vi "validate inputs.vi"(9 "output in":T5, 10 "process in":T3, 11 "input in":T4) -> (3 "spec":T1[](array[typedef]))   [LabVIEW 2013, in "data interface script.lvlib"]
uses:
  data interface script.lvlib
  Controls/output script control.ctl
  Controls/input script control.ctl
  Controls/processing script control.ctl
  Controls/scripting spec.ctl
  <vilib>/NI/Tag Bus Module Framework/channel/channel classification.ctl
  <vilib>/NI/Tag Bus Module Framework/channel/TBM channel.lvclass
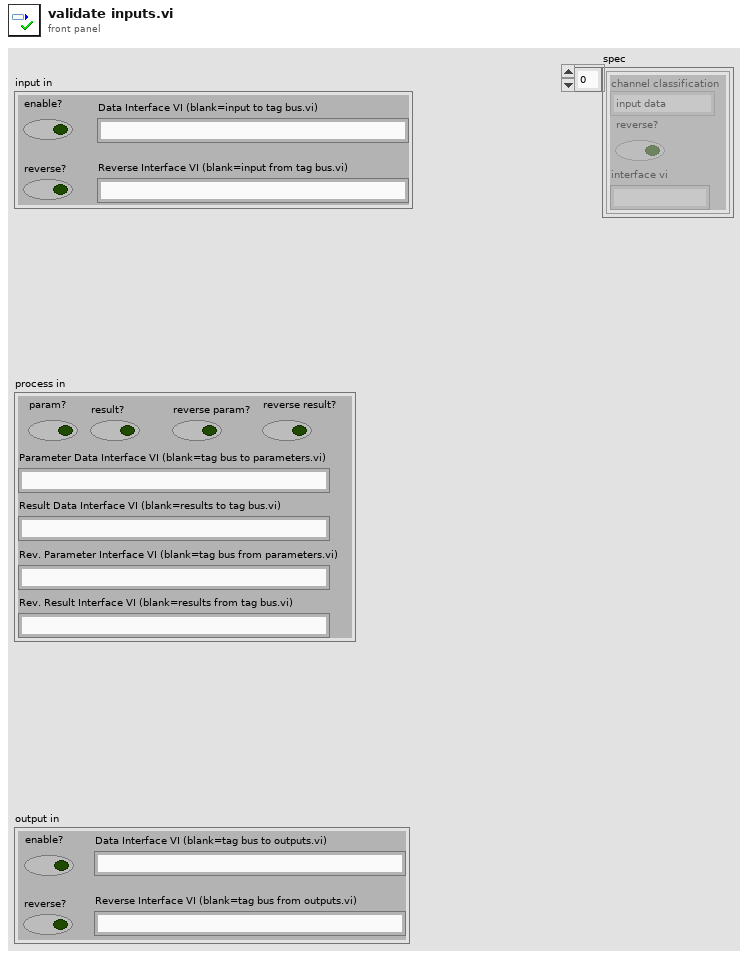
[diagram p1: front panel]
types:
  T1 = typedef "data interface script.lvlib/scripting spec.ctl" = cluster{"channel classification":T2, "reverse?":bool, "interface vi":string}
  T2 = typedef "TBM channel.lvclass/channel classification.ctl" = enum16{"input data", "output data", "processing parameter", "processing result"}
  T3 = typedef "data interface script.lvlib/processing script control.ctl" = cluster{"param?":bool, "Parameter Data Interface VI (blank=tag bus to parameters.vi)":string, "Result Data Interface VI (blank=results to tag bus.vi)":string, "reverse param?":bool, "Rev. Result Interface VI (blank=results from tag bus.vi)":string, "Rev. Parameter Interface VI (blank=tag bus from parameters.vi)":string, "result?":bool, "reverse result?":bool}
  T4 = typedef "data interface script.lvlib/input script control.ctl" = cluster{"enable?":bool, "Data Interface VI (blank=input to tag bus.vi)":string, "reverse?":bool, "Reverse Interface VI (blank=input from tag bus.vi)":string}
  T5 = typedef "data interface script.lvlib/output script control.ctl" = cluster{"enable?":bool, "Data Interface VI (blank=tag bus to outputs.vi)":string, "Reverse Interface VI (blank=tag bus from outputs.vi)":string, "reverse?":bool}
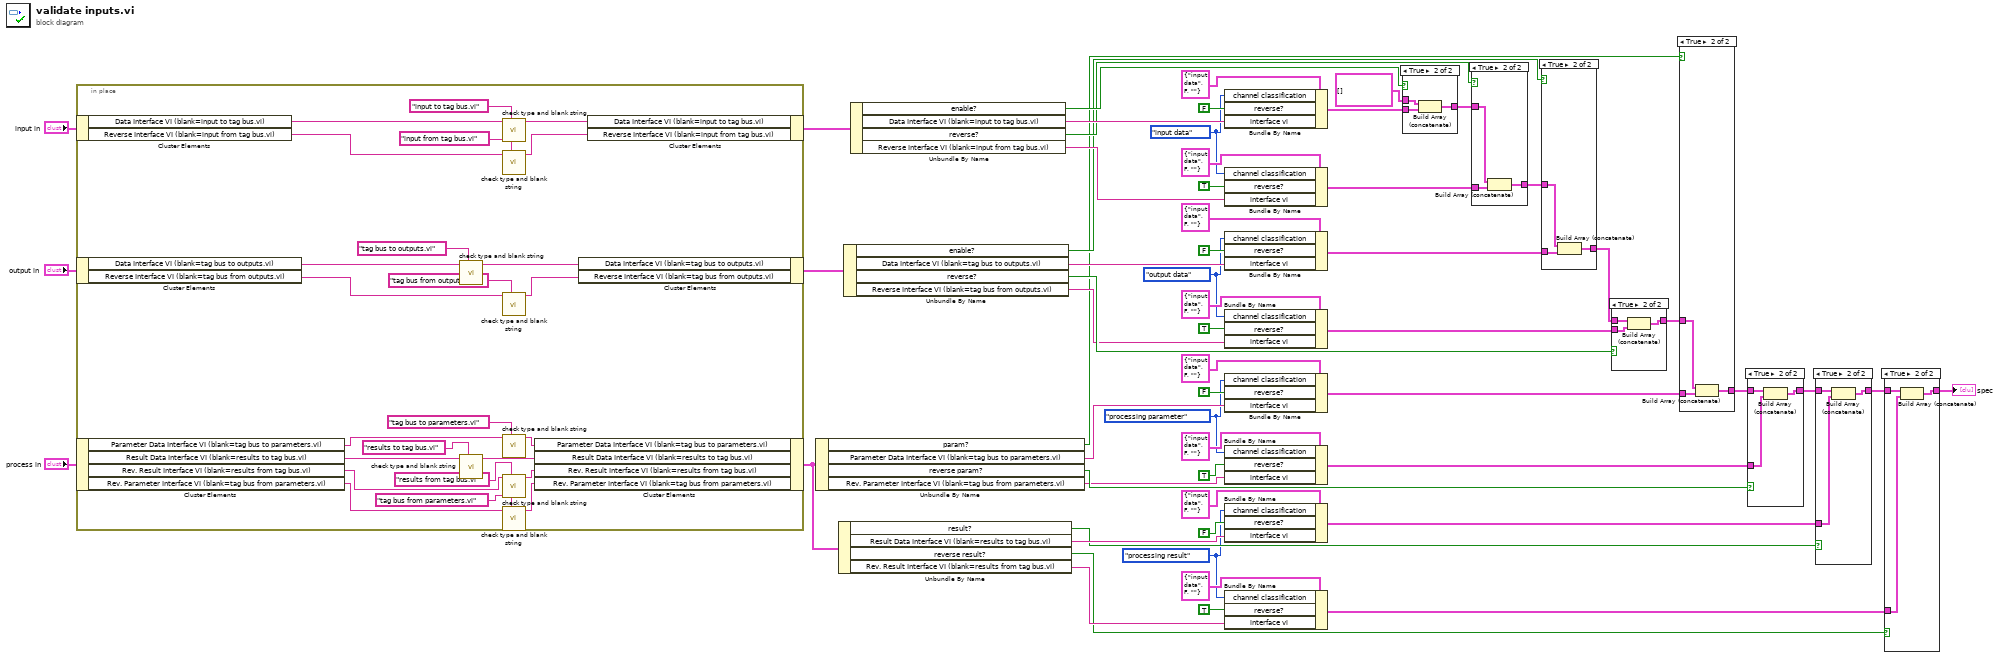
[diagram p0: block diagram]
diagram:
  w2 = channel_classification."processing result" ("channel classification")
  w3 = channel_classification."processing parameter" ("channel classification")
  w5 = channel_classification."output data" ("channel classification")
  w4 = channel_classification."input data" ("channel classification")
  n1 = in-place {
    n2 = in-place-cluster #1("input in") -> ("Data Interface VI (blank=input to tag bus.vi)"=w82:string, "Reverse Interface VI (blank=input from tag bus.vi)"=w69:string)
    n3 = in-place-cluster #2("output in") -> ("Data Interface VI (blank=tag bus to outputs.vi)"=w80:string, "Reverse Interface VI (blank=tag bus from outputs.vi)"=w61:string)
    n4 = in-place-cluster #3("process in") -> ("Parameter Data Interface VI (blank=tag bus to parameters.vi)"=w77:string, "Result Data Interface VI (blank=results to tag bus.vi)"=w76:string, "Rev. Result Interface VI (blank=results from tag bus.vi)"=w66:string, "Rev. Parameter Interface VI (blank=tag bus from parameters.vi)"=w63:string)
    n5 = call "check type and blank string.vi"("default"="tag bus to outputs.vi", "user input"=w80) -> ("validated"=w81:string)  [unwired: 9 in]
    n6 = call "check type and blank string.vi"("default"="results to tag bus.vi", "user input"=w76) -> ("validated"=w79:string)  [unwired: 9 in]
    n7 = call "check type and blank string.vi"("default"="input to tag bus.vi", "user input"=w82) -> ("validated"=w83:string)  [unwired: 9 in]
    n8 = call "check type and blank string.vi"("default"="input from tag bus.vi", "user input"=w69) -> ("validated"=w70:string)  [unwired: 9 in]
    n9 = call "check type and blank string.vi"("default"="tag bus from outputs.vi", "user input"=w61) -> ("validated"=w60:string)  [unwired: 9 in]
    n10 = call "check type and blank string.vi"("default"="tag bus to parameters.vi", "user input"=w77) -> ("validated"=w78:string)  [unwired: 9 in]
    n11 = call "check type and blank string.vi"("default"="results from tag bus.vi", "user input"=w66) -> ("validated"=w65:string)  [unwired: 9 in]
    n12 = call "check type and blank string.vi"("default"="tag bus from parameters.vi", "user input"=w63) -> ("validated"=w64:string)  [unwired: 9 in]
    n13 = in-place-cluster #3("Parameter Data Interface VI (blank=tag bus to parameters.vi)"=w78, "Result Data Interface VI (blank=results to tag bus.vi)"=w79, "Rev. Result Interface VI (blank=results from tag bus.vi)"=w65, "Rev. Parameter Interface VI (blank=tag bus from parameters.vi)"=w64) -> (w6:T3)
    n14 = in-place-cluster #2("Data Interface VI (blank=tag bus to outputs.vi)"=w81, "Reverse Interface VI (blank=tag bus from outputs.vi)"=w60) -> (w31:T5)
    n15 = in-place-cluster #1("Data Interface VI (blank=input to tag bus.vi)"=w83, "Reverse Interface VI (blank=input from tag bus.vi)"=w70) -> (w56:T4)
  }
  n16 = Unbundle By Name(w6) -> ("param?"=w14:bool, "Parameter Data Interface VI (blank=tag bus to parameters.vi)"=w9:string, "reverse param?"=w18:bool, "Rev. Parameter Interface VI (blank=tag bus from parameters.vi)"=w13:string)
  n17 = Unbundle By Name(w6) -> ("result?"=w23:bool, "Result Data Interface VI (blank=results to tag bus.vi)"=w28:string, "reverse result?"=w19:bool, "Rev. Result Interface VI (blank=results from tag bus.vi)"=w24:string)
  n18 = Unbundle By Name(w31) -> ("enable?"=w39:bool, "Data Interface VI (blank=tag bus to outputs.vi)"=w34:string, "reverse?"=w43:bool, "Reverse Interface VI (blank=tag bus from outputs.vi)"=w38:string)
  n19 = Unbundle By Name(w56) -> ("enable?"=w49:bool, "Data Interface VI (blank=input to tag bus.vi)"=w54:string, "reverse?"=w44:bool, "Reverse Interface VI (blank=input from tag bus.vi)"=w50:string)
  n20 = Bundle By Name(cluster=T1 {"channel classification"=enum."input data", "reverse?"=FALSE, "interface vi"=""} ("spec"), "channel classification"=w4, "reverse?"=FALSE, "interface vi"=w54) -> (w48:T1)
  n21 = Bundle By Name(cluster=T1 {"channel classification"=enum."input data", "reverse?"=FALSE, "interface vi"=""} ("spec"), "channel classification"=w4, "reverse?"=TRUE, "interface vi"=w50) -> (w45:T1)
  n22 = Bundle By Name(cluster=T1 {"channel classification"=enum."input data", "reverse?"=FALSE, "interface vi"=""} ("spec"), "channel classification"=w5, "reverse?"=FALSE, "interface vi"=w34) -> (w40:T1)
  n23 = Bundle By Name(cluster=T1 {"channel classification"=enum."input data", "reverse?"=FALSE, "interface vi"=""} ("spec"), "channel classification"=w5, "reverse?"=TRUE, "interface vi"=w38) -> (w42:T1)
  n24 = Bundle By Name(cluster=T1 {"channel classification"=enum."input data", "reverse?"=FALSE, "interface vi"=""} ("spec"), "channel classification"=w3, "reverse?"=FALSE, "interface vi"=w9) -> (w15:T1)
  n25 = Bundle By Name(cluster=T1 {"channel classification"=enum."input data", "reverse?"=FALSE, "interface vi"=""} ("spec"), "channel classification"=w3, "reverse?"=TRUE, "interface vi"=w13) -> (w17:T1)
  n26 = Bundle By Name(cluster=T1 {"channel classification"=enum."input data", "reverse?"=FALSE, "interface vi"=""} ("spec"), "channel classification"=w2, "reverse?"=FALSE, "interface vi"=w28) -> (w22:T1)
  n27 = Bundle By Name(cluster=T1 {"channel classification"=enum."input data", "reverse?"=FALSE, "interface vi"=""} ("spec"), "channel classification"=w2, "reverse?"=TRUE, "interface vi"=w24) -> (w20:T1)
  n28 = case shown="True" w49 {
    tunnel: w48 -> [_ w87]
    tunnel: T1[] [] -> [w84 w86]
    tunnel: [w84 w85] -> w46
    frame False {
    }
    frame True {
      n29 = Build Array (concatenate)(w86, w87) -> (w85:T1[])
    }
  }
  n30 = case shown="True" w44 {
    tunnel: w45 -> [_ w91]
    tunnel: w46 -> [w88 w90]
    tunnel: [w88 w89] -> w32
    frame False {
    }
    frame True {
      n31 = Build Array (concatenate)(w90, w91) -> (w89:T1[])
    }
  }
  n32 = case shown="True" w39 {
    tunnel: w40 -> [_ w95]
    tunnel: w32 -> [w92 w94]
    tunnel: [w92 w93] -> w41
    frame False {
    }
    frame True {
      n33 = Build Array (concatenate)(w94, w95) -> (w93:T1[])
    }
  }
  n34 = case shown="True" w43 {
    tunnel: w42 -> [_ w99]
    tunnel: w41 -> [w96 w98]
    tunnel: [w96 w97] -> w7
    frame False {
    }
    frame True {
      n35 = Build Array (concatenate)(w98, w99) -> (w97:T1[])
    }
  }
  n36 = case shown="True" w14 {
    tunnel: w15 -> [_ w103]
    tunnel: w7 -> [w100 w102]
    tunnel: [w100 w101] -> w16
    frame False {
    }
    frame True {
      n37 = Build Array (concatenate)(w102, w103) -> (w101:T1[])
    }
  }
  n38 = case shown="True" w18 {
    tunnel: w17 -> [_ w107]
    tunnel: w16 -> [w104 w106]
    tunnel: [w104 w105] -> w30
    frame False {
    }
    frame True {
      n39 = Build Array (concatenate)(w106, w107) -> (w105:T1[])
    }
  }
  n40 = case shown="True" w23 {
    tunnel: w22 -> [_ w111]
    tunnel: w30 -> [w108 w110]
    tunnel: [w108 w109] -> w21
    frame False {
    }
    frame True {
      n41 = Build Array (concatenate)(w110, w111) -> (w109:T1[])
    }
  }
  n42 = case shown="True" w19 {
    tunnel: w20 -> [_ w115]
    tunnel: w21 -> [w112 w114]
    tunnel: [w112 w113] -> w1
    frame False {
    }
    frame True {
      n43 = Build Array (concatenate)(w114, w115) -> (w113:T1[])
    }
  }
  "spec" <- w1
